vi "Add Default Enum.vi"(6 "Hdr Name":T1, 8 "error in (no error)":errorcluster, 9 "Enum Values":u16[](array[numeric]), 11 "RTD in":refnum<class "RTD.lvclass">) -> (0 "error out":errorcluster, 3 "RTD out":refnum<class "RTD.lvclass">)   [LabVIEW 2012, in "Measurement Channels.lvlib" / "RTD.lvclass"]
uses:
  RTD.lvclass
  Common/Controls/HeaderNames.ctl
  RTD.lvclass/RTD.ctl
  SubVIs Table/Custom Ctls Table/ge_ColType.ctl
  Class Channel/Write Unit_EU.vi
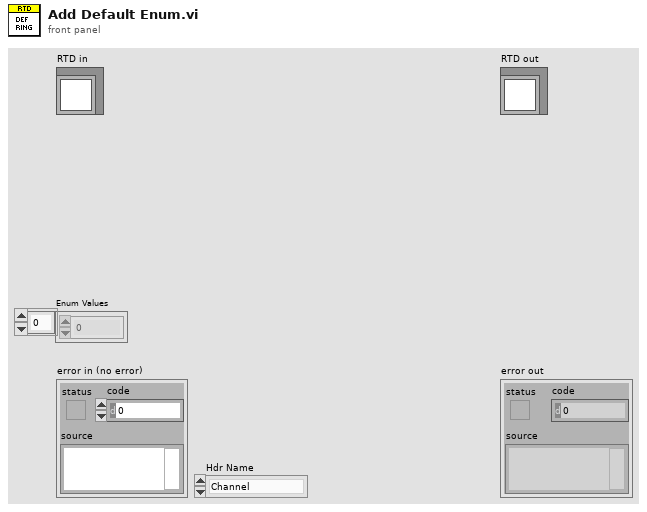
[diagram p1: front panel]
types:
  T1 = typedef "HeaderNames.ctl" = enum16{"Channel", "Device", "Spacer", "Description", "MB", "Range", "Terminal", "Coupling", "Thresh (V)", "Pulse/Rev", "Slope", "Min EU", "Min RPM", "mV/EU", "Iex", "Temp Units", "Type", "CJC Src", "CJC Val", "Ro", "Wire Cfg", "Strain Mode", "Vex", "Bridge Type", "GF", "Gauge Res", "Poisson", "Lead Res", "Init Strain", "GAF", "Scale", "Offset", "Unit (EU)", "dB?", "dB Ref", "Cal Mag", "Cal Units", "Max Temp", "Min Temp", "Max Strain", "Min Strain"}
  T2 = typedef "ge_ColType.ctl" = enum16{"Volts", "Amps", "Ohms", "TermCfg", "WireCfg", "Coup", "Slope", "Iex", "CalUnits", "ThrmUnits", "ThrmType", "CJCSrc", "BrdgType", "Strn Mode", "RTDType"}
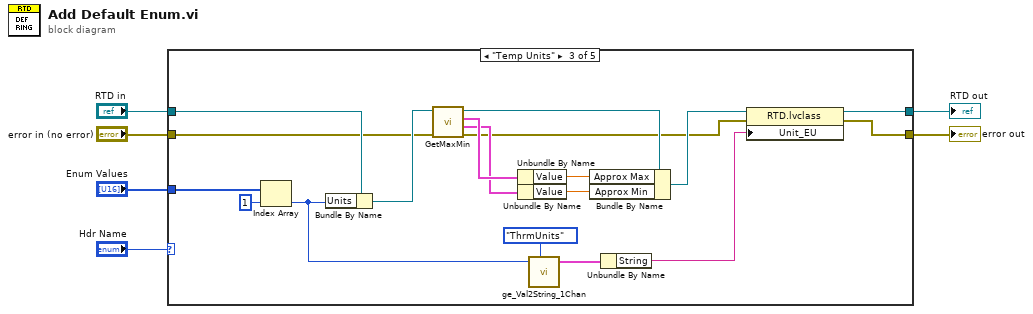
[diagram p0: block diagram]
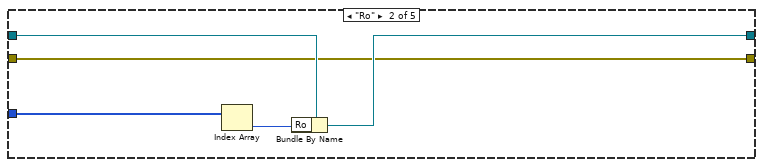
[diagram p3: hidden frame]
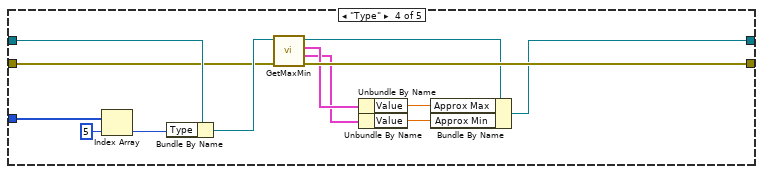
[diagram p4: hidden frame]
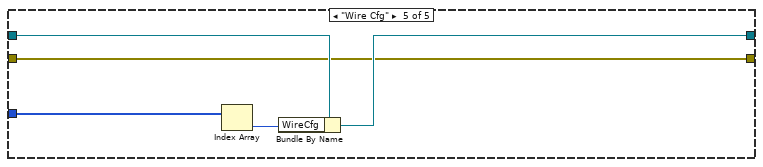
[diagram p5: hidden frame]
diagram:
  n1 = case shown="\"Temp Units\"" "Hdr Name" {
    tunnel: "RTD in" -> [w8 w13 w31 w44 w49]
    tunnel: "error in (no error)" -> [w7 w9 w29 w42 w45]
    tunnel: [w8 w10 w21 w38 w46] -> w2
    tunnel: [w7 w9 w19 w41 w45] -> w1
    tunnel: "Enum Values" -> [_ w11 w23 w33 w47]
    frame Default {
    }
    frame "Ro" {
      n2 = Index Array(array=w11) -> (element=w12:u16)  [unwired: 1 in]
      n3 = Bundle By Name(cluster=w13, "Ro"=w12) -> (w10:refnum<class "RTD.lvclass">)
    }
    frame "Temp Units" {
      n4 = Index Array(array=w23, index=1) -> (element=w15:u16)
      n5 = Bundle By Name(cluster=w31, "Units"=w15) -> (w30:refnum<class "RTD.lvclass">)
      n6 = call-dynamic "GetMaxMin.vi"("error in (no error)"=w29, "RTD in"=w30) -> ("error out"=w18:errorcluster, "Min"=w24:cluster{"Value":dbl, "Text":string}, "Max"=w27:cluster{"Value":dbl, "Text":string}, "RTD out"=w28:refnum<class "RTD.lvclass">)  [unwired: 6 in]
      n7 = Unbundle By Name(w27) -> ("Value"=w26:dbl)
      n8 = Unbundle By Name(w24) -> ("Value"=w25:dbl)
      n9 = call "ge_Val2String_1Chan.vi"("Value"=w15, "ColType"=ge_ColType."ThrmUnits") -> ("String and Val"=w16:cluster{"String":string, "Value":u16})  [unwired: 5 in]
      n10 = Bundle By Name(cluster=w28, "Approx Max"=w26, "Approx Min"=w25) -> (w20:refnum<class "RTD.lvclass">)
      n11 = Unbundle By Name(w16) -> ("String"=w14:string)
      n12 = property class="RTD.lvclass"(reference=w20, error in=w18, "Unit_EU"=w14) -> (reference out=w21:refnum<class "RTD.lvclass">, error out=w19:errorcluster)
    }
    frame "Type" {
      n13 = Index Array(array=w33, index=5) -> (element=w40:u16)
      n14 = Bundle By Name(cluster=w44, "Type"=w40) -> (w43:refnum<class "RTD.lvclass">)
      n15 = call-dynamic "GetMaxMin.vi"("error in (no error)"=w42, "RTD in"=w43) -> ("error out"=w41:errorcluster, "Min"=w34:cluster{"Value":dbl, "Text":string}, "Max"=w37:cluster{"Value":dbl, "Text":string}, "RTD out"=w39:refnum<class "RTD.lvclass">)  [unwired: 6 in]
      n16 = Unbundle By Name(w37) -> ("Value"=w36:dbl)
      n17 = Unbundle By Name(w34) -> ("Value"=w35:dbl)
      n18 = Bundle By Name(cluster=w39, "Approx Max"=w36, "Approx Min"=w35) -> (w38:refnum<class "RTD.lvclass">)
    }
    frame "Wire Cfg" {
      n19 = Index Array(array=w47) -> (element=w48:u16)  [unwired: 1 in]
      n20 = Bundle By Name(cluster=w49, "WireCfg"=w48) -> (w46:refnum<class "RTD.lvclass">)
    }
  }
  "error out" <- w1
  "RTD out" <- w2
